vi "Cancel State Machine - Load.vi"   [LabVIEW 2013]
uses:
  typedefs/State Machine/subStates.ctl
  typedefs/fg_typedef.ctl
  typedefs/DevRef Type.ctl
  typedefs/State Machine/singleUseSubstate.ctl
  <vilib>/Rock Robotics/WPI/Solenoid/WPI_SolenoidValue.ctl
  <vilib>/Rock Robotics/WPI/Solenoid/WPI_SolenoidGetEnum.vi
panel:
  # "A State Machine to Handle Canceling Load"
types:
  T1 = typedef "subStates.ctl" = enum16{"null", "wait", "driver control", "auto", "manual override", "hold position", "rotate", "pickup", "pass", "recover pass", "load", "goto shoot", "shoot high goal", "shoot low goal", "cancel arm", "cancel shooter", "end", "test"}
  T2 = typedef "DevRef Type.ctl" = enum16{"Shooter Solenoid", "Latch Solenoid", "Right Up Sensor", "Right Down Sensor", "Hold Sensor", "Arm Encoder"}
  T3 = typedef "fg_typedef.ctl" = enum16{"Get", "Set"}
  T4 = typedef "WPI_SolenoidValue.ctl" = enum16{"Off", "On", "Forward", "Reverse"}
  T5 = typedef "singleUseSubstate.ctl" = enum16{"null", "wait", "shift high", "shift low", "extend shooter", "retract shooter", "latch", "unlatch", "end"}
  T6 = typedef "WPI_EncoderDevRef.ctl" = cluster{"DevStatus":errorcluster, "EncoderIndex":T7, "CounterIndex":T8, "DistancePerCount":dbl, "Decoding Type":T9}
  T7 = typedef "FPGA_EncoderIdx.ctl" = enum8{"Enc 0", "Enc 1", "Enc 2", "Enc 3", "Invalid"}
  T8 = typedef "FPGA_CounterCtrSystemIndex.ctl" = enum8{"Ctr 0", "Ctr 1", "Ctr 2", "Ctr 3", "Ctr 4", "Ctr 5", "Ctr 6", "Ctr 7", "Invalid"}
  T9 = typedef "WPI_EncoderType.ctl" = enum16{"1x", "2x", "4x"}
  T10 = typedef "WPI_DigitalInputDevRef.ctl" = cluster{"DevStatus":errorcluster, "DIO Channel":T11, "Digital Module":T12}
  T11 = typedef "FPGA_DIOChannel.ctl" = enum8{"DIO 1", "DIO 2", "DIO 3", "DIO 4", "DIO 5", "DIO 6", "DIO 7", "DIO 8", "DIO 9", "DIO 10", "DIO 11", "DIO 12", "DIO 13", "DIO 14", "Invalid"}
  T12 = typedef "FPGA_TypedefDigitalModule.ctl" = enum16{"Digital Module 1", "Digital Module 2"}
  T13 = typedef "WPI_SolenoidDevRef.ctl" = cluster{"DevStatus":errorcluster, "Solenoid Module":T14, "Forward Solenoid Channel":T15, "Reverse Solenoid Channel":T15}
  T14 = typedef "FPGA_TypedefSolenoidModule.ctl" = enum16{"Solenoid Module 1", "Solenoid Module 2"}
  T15 = typedef "WPI_SolenoidChannel.ctl" = enum8{"Solenoid 1", "Solenoid 2", "Solenoid 3", "Solenoid 4", "Solenoid 5", "Solenoid 6", "Solenoid 7", "Solenoid 8", "Invalid"}
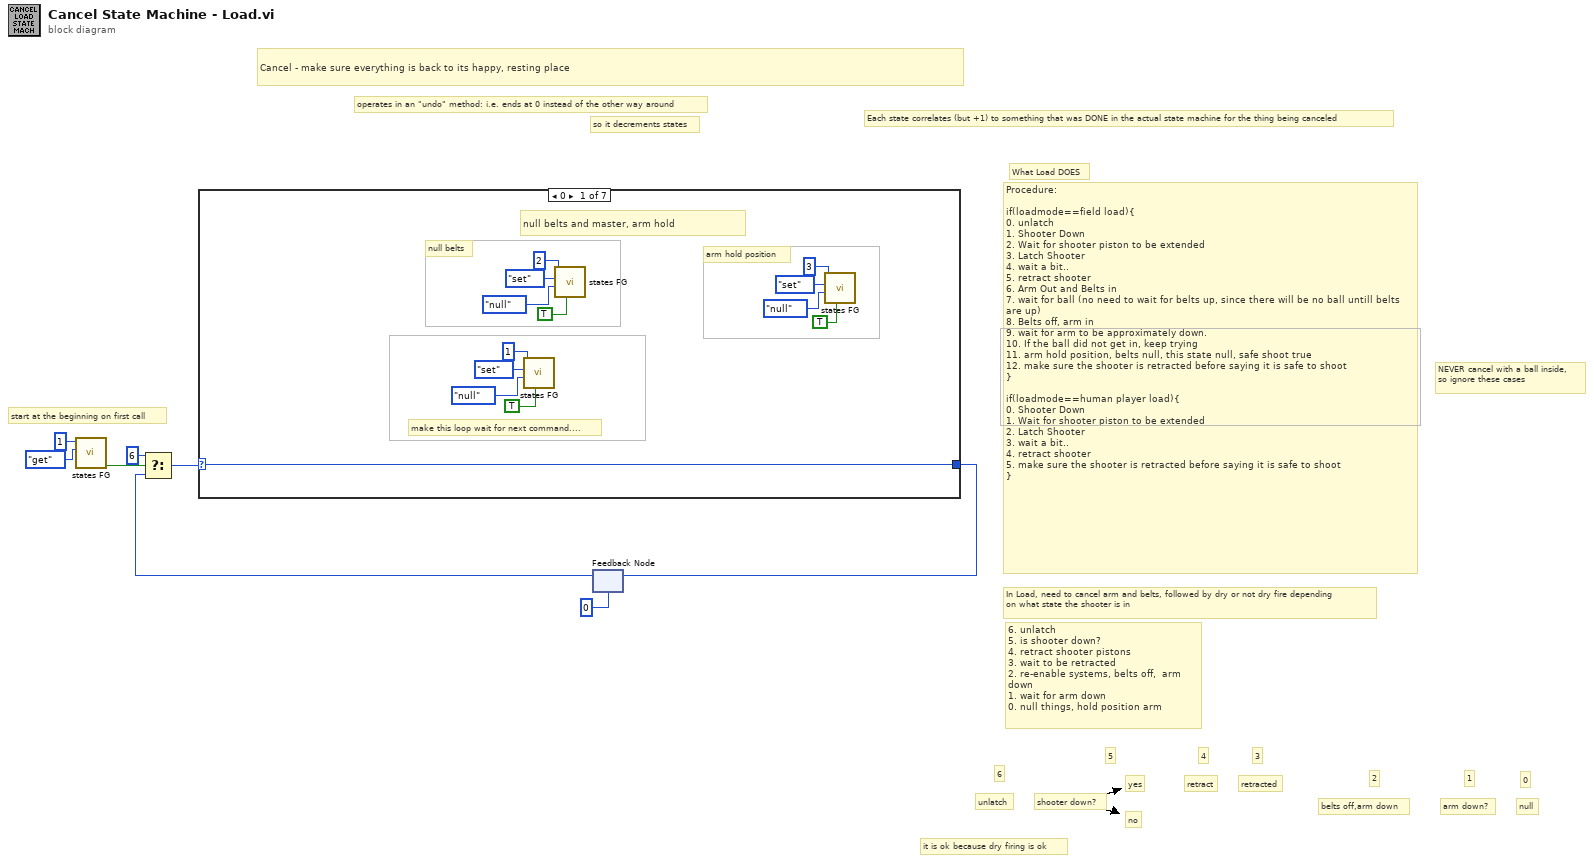
[diagram p0: block diagram]
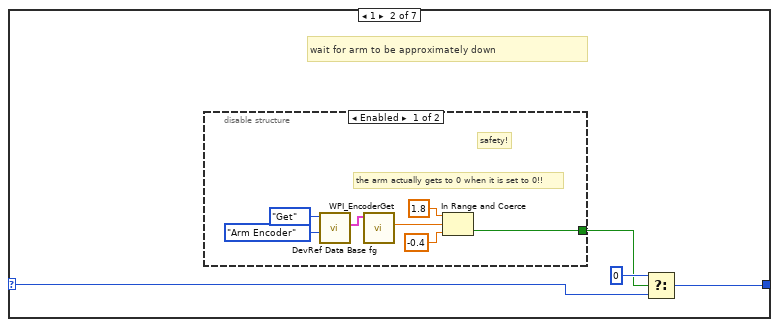
[diagram p2: hidden frame]
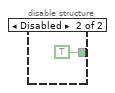
[diagram p3: hidden frame]
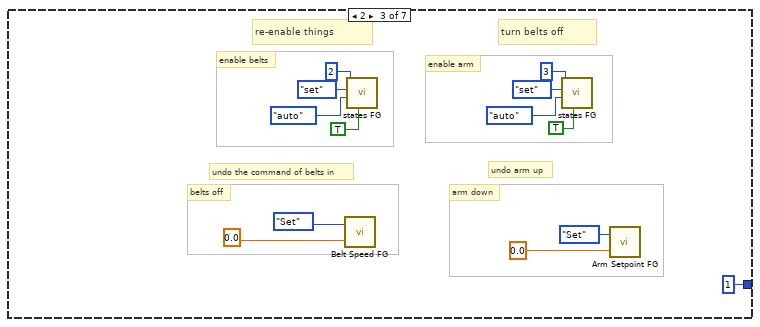
[diagram p4: hidden frame]
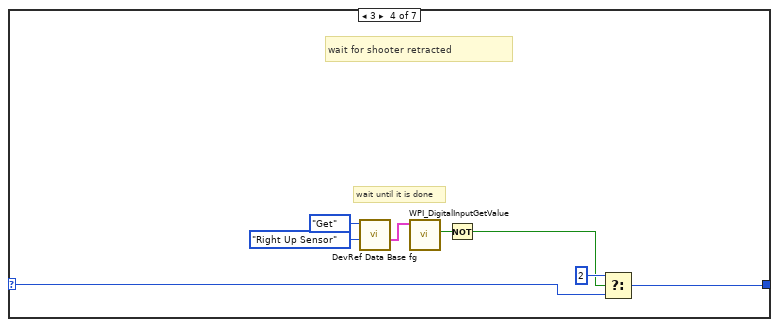
[diagram p5: hidden frame]
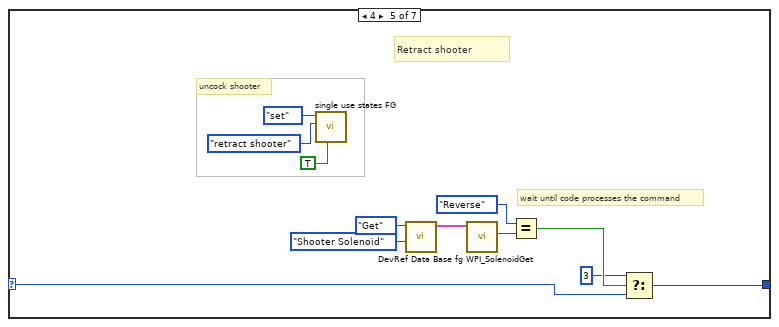
[diagram p6: hidden frame]
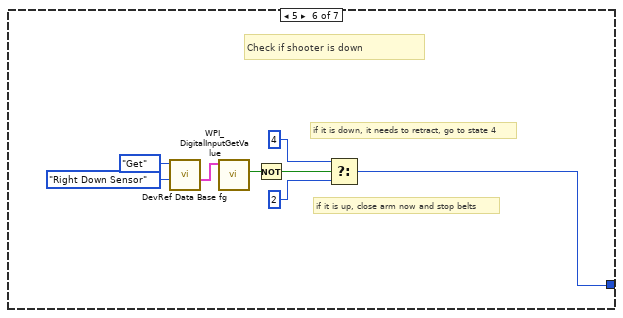
[diagram p7: hidden frame]
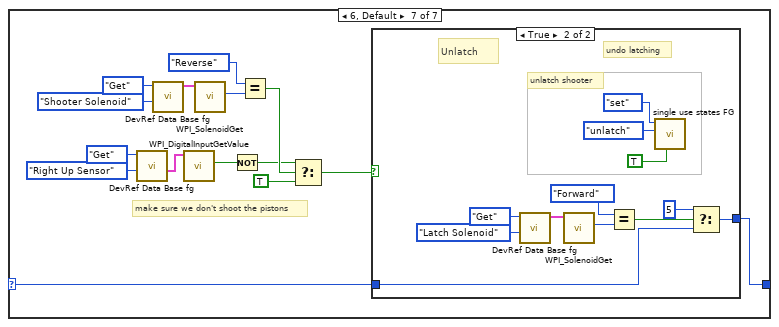
[diagram p8: hidden frame]
diagram:
  # "3"
  # "retracted"
  # "1"
  # "arm down?"
  # "it is ok because dry firing is ok"
  # "0"
  # "4"
  # "5"
  # "6"
  # "2"
  # "null"
  # "unlatch"
  # "retract"
  # "no"
  # "yes"
  # "shooter down?"
  # "belts off,arm down"
  # "NEVER cancel with a ball inside,\nso ignore these cases"
  # "What Load DOES"
  # "so it decrements states"
  # "Each state correlates (but +1) to something that was DONE in the actual state machine for the thing being canceled"
  # "6. unlatch\n5. is shooter down?\n4. retract shooter pistons\n3. wait to be retracted\n2. re-enable systems, belts off,  arm down\n1. wait for arm down\n0. null things, hold position arm"
  # "In Load, need to cancel arm and belts, followed by dry or not dry fire depending\non what state the shooter is in"
  # "operates in an \"undo\" method: i.e. ends at 0 instead of the other way around"
  # "start at the beginning on first call"
  # "Cancel - make sure everything is back to its happy, resting place"
  # "Procedure: \n\nif(loadmode==field load){\n0. unlatch\n1. Shooter Down \n2. Wait for shooter piston to be extended\n3. Latch Shooter\n4. wait a bit..\n5. retract shooter\n6. Arm Out and Belts in\n7. wait for ball (no need to wait for belts up, since there will be no ball untill belts are up)\n8. Belts off, arm in\n9. wait for arm to be approximately down.\n10. If the ball did not get in, keep trying\n11. arm hold position, belts null, this state null, safe shoot true\n12. make sure the shooter is retracted before saying it is safe to shoot\n}\n\nif(loadmode==human player load){\n0. Shooter Down \n1. Wait for shooter piston to be extended\n2. Latch Shooter\n3. wait a bit..\n4. retract shooter\n5. make sure the shooter is retracted before saying it is safe to shoot\n}"
  n1 = call "states FG.vi"("menu (get)"=enum16{"set", "get"}."get", "Loop ID"=1) -> ("first call?"=w8:bool)  [unwired: 6 in, 3 out]
  n2 = feedback #1(u8 0) -> (w3:u8)
  n3 = Select(t=u8 6, s=w8, f=w3) -> (s? t:f=w5:u8)
  n4 = case shown="0" w5 {
    selector: w5 -> [w21 w25 _ w52 w63 _ w89]
    tunnel: [w21 w24 u8 1 ("t") w51 w62 w71 w88] -> w2
    frame 0 {
      # "null belts and master, arm hold"
      # "make this loop wait for next command...."
      # "arm hold position"
      # "null belts"
      n5 = call "states FG.vi"("exit in"=TRUE, "subState in"=subStates."null", "menu (get)"=enum16{"set", "get"}."set", "Loop ID"=1) -> ()  [unwired: 4 in, 4 out]
      n6 = call "states FG.vi"("exit in"=TRUE, "subState in"=subStates."null", "menu (get)"=enum16{"set", "get"}."set", "Loop ID"=2) -> ()  [unwired: 4 in, 4 out]
      n7 = call "states FG.vi"("exit in"=TRUE, "subState in"=subStates."null", "menu (get)"=enum16{"set", "get"}."set", "Loop ID"=3) -> ()  [unwired: 4 in, 4 out]
    }
    frame 1 {
      # "wait for arm to be approximately down"
      n8 = disable-structure shown="Enabled" {
        disable-tunnel: [w28 TRUE] -> w22
        frame Enabled {
          # "safety!"
          # "the arm actually gets to 0 when it is set to 0!!"
          n9 = call "DevRef Data Base fg.vi"("DevRef to Get"=DevRef_Type."Arm Encoder", "Menu"=fg_typedef."Get") -> ("Selected Encoder"=w32:T6)  [unwired: 1 in, 8 out]
          n10 = call <vilib>:"WPI_EncoderGet.vi"("EncoderDevRef"=w32) -> ("Distance"=w31:dbl)  [unwired: 5 in, 5 out]
          n11 = In Range and Coerce(upper limit=1.8, x=w31, lower limit=-0.4 ("upper limit")) -> (In Range?=w28:bool)  [unwired: 1 out]
        }
        frame Disabled {
        }
      }
      n12 = Select(t=u8 0, s=w22, f=w25) -> (s? t:f=w24:u8)
    }
    frame 2 {
      # "undo arm up"
      # "arm down"
      # "re-enable things"
      # "turn belts off"
      # "undo the command of belts in"
      # "belts off"
      # "enable arm"
      # "enable belts"
      n13 = call "Belt Speed FG.vi"("Speed In"=0.0 ("Setpoint In"), "Menu"=fg_typedef."Set") -> ()  [unwired: 1 out]
      n14 = call "states FG.vi"("exit in"=TRUE, "subState in"=subStates."auto", "menu (get)"=enum16{"set", "get"}."set", "Loop ID"=2) -> ()  [unwired: 4 in, 4 out]
      n15 = call "states FG.vi"("exit in"=TRUE, "subState in"=subStates."auto", "menu (get)"=enum16{"set", "get"}."set", "Loop ID"=3) -> ()  [unwired: 4 in, 4 out]
      n16 = call "Arm Setpoint FG.vi"("Setpoint In"=0.0, "Menu"=fg_typedef."Set") -> ()  [unwired: 1 out]
    }
    frame 3 {
      # "wait until it is done"
      # "wait for shooter retracted"
      n17 = call "DevRef Data Base fg.vi"("DevRef to Get"=DevRef_Type."Right Up Sensor", "Menu"=fg_typedef."Get") -> ("Selected Sensor"=w53:T10)  [unwired: 1 in, 8 out]
      n18 = call <vilib>:"WPI_DigitalInputGetValue.vi"("DigitalInputDevRef"=w53) -> ("Value"=w54:bool)  [unwired: 8 in, 2 out]
      n19 = Not(x=w54) -> (.not. x?=w49:bool)
      n20 = Select(t=u8 2, s=w49, f=w52) -> (s? t:f=w51:u8)
    }
    frame 4 {
      # "wait until code processes the command"
      # "uncock shooter"
      # "Retract shooter"
      n21 = call "single use states FG.vi"("exit in"=TRUE, "substate"=singleUseSubstate."retract shooter", "menu (get)"=enum16{"set", "get"}."set") -> ()  [unwired: 5 in, 4 out]
      n22 = call "DevRef Data Base fg.vi"("DevRef to Get"=DevRef_Type."Shooter Solenoid", "Menu"=fg_typedef."Get") -> ("Selected Solenoid"=w61:T13)  [unwired: 1 in, 8 out]
      n23 = call-poly <vilib>:"WPI_SolenoidGet.vi"("SolenoidDevRef"=w61) -> ("Value"=w60:T4)  [unwired: 8 in, 2 out]
      n24 = Equal?(x=WPI_SolenoidValue."Reverse", y=w60) -> (x = y?=w58:bool)
      n25 = Select(t=u8 3, s=w58, f=w63) -> (s? t:f=w62:u8)
    }
    frame 5 {
      # "if it is up, close arm now and stop belts"
      # "if it is down, it needs to retract, go to state 4"
      # "Check if shooter is down"
      n26 = call "DevRef Data Base fg.vi"("DevRef to Get"=DevRef_Type."Right Down Sensor", "Menu"=fg_typedef."Get") -> ("Selected Sensor"=w73:T10)  [unwired: 1 in, 8 out]
      n27 = call <vilib>:"WPI_DigitalInputGetValue.vi"("DigitalInputDevRef"=w73) -> ("Value"=w74:bool)  [unwired: 8 in, 2 out]
      n28 = Not(x=w74) -> (.not. x?=w72:bool)
      n29 = Select(t=u8 4, s=w72, f=u8 2) -> (s? t:f=w71:u8)
    }
    frame 6, Default {
      # "make sure we don't shoot the pistons"
      n30 = call "DevRef Data Base fg.vi"("DevRef to Get"=DevRef_Type."Right Up Sensor", "Menu"=fg_typedef."Get") -> ("Selected Sensor"=w78:T10)  [unwired: 1 in, 8 out]
      n31 = call "DevRef Data Base fg.vi"("DevRef to Get"=DevRef_Type."Shooter Solenoid", "Menu"=fg_typedef."Get") -> ("Selected Solenoid"=w85:T13)  [unwired: 1 in, 8 out]
      n32 = call <vilib>:"WPI_DigitalInputGetValue.vi"("DigitalInputDevRef"=w78) -> ("Value"=w77:bool)  [unwired: 8 in, 2 out]
      n33 = call-poly <vilib>:"WPI_SolenoidGet.vi"("SolenoidDevRef"=w85) -> ("Value"=w83:T4)  [unwired: 8 in, 2 out]
      n34 = Not(x=w77) -> (.not. x?=w76:bool)
      n35 = Equal?(x=WPI_SolenoidValue."Reverse" ("Value"), y=w83) -> (x = y?=w82:bool)
      n36 = Select(t=w76, s=w82, f=TRUE) -> (s? t:f=w75:bool)
      n37 = case shown="True" w75 {
        tunnel: w89 -> [w90 w95]
        tunnel: [w90 w94] -> w88
        frame False {
        }
        frame True {
          # "unlatch shooter"
          # "undo latching"
          # "Unlatch"
          n38 = call "DevRef Data Base fg.vi"("DevRef to Get"=DevRef_Type."Latch Solenoid", "Menu"=fg_typedef."Get") -> ("Selected Solenoid"=w99:T13)  [unwired: 1 in, 8 out]
          n39 = call-poly <vilib>:"WPI_SolenoidGet.vi"("SolenoidDevRef"=w99) -> ("Value"=w97:T4)  [unwired: 8 in, 2 out]
          n40 = Equal?(x=WPI_SolenoidValue."Forward" ("Value"), y=w97) -> (x = y?=w96:bool)
          n41 = call "single use states FG.vi"("exit in"=TRUE, "substate"=singleUseSubstate."unlatch", "menu (get)"=enum16{"set", "get"}."set") -> ()  [unwired: 5 in, 4 out]
          n42 = Select(t=u8 5, s=w96, f=w95) -> (s? t:f=w94:u8)
        }
      }
    }
  }
  n43 = feedback-in #1(w2) -> ()
